vi "Configure Digital Alarm Parameters.vi"(0 "VISA resource name":refnum<visa-resource-name>, 1 "Alarm Number (1)":u16=1 min=1 max=8, 2 "Unit Address (1)":u8=1, 5 "Latching Mode (0: No Latch)":u16(ring)=1 items=["No Latch", "Automatic Latching", "Manual Latching", "Event Latching"], 7 "Priority (1: Low Priority)":u8(ring)=1 items=["Low Priority"=1, "Medium Priority"=2, "High Priority"=3], 9 "Display Delay (0)":u32 max=1800000000, 11 "error in (no error)":errorcluster, 12 "Alarm Inhibit  (False: Disable)":bool, 13 "Alarm Blocking Mode (False: Disable)":bool) -> (4 "VISA resource name out":refnum<visa-resource-name>, 15 "error out":errorcluster)   [LabVIEW 2014, in "Eurotherm 35xx Series.lvlib"]
doc: "This VI Configure parameters of selected digital alarm."
uses:
  <instrlib>/Eurotherm 35xx Series/Eurotherm 35xx Series.lvlib
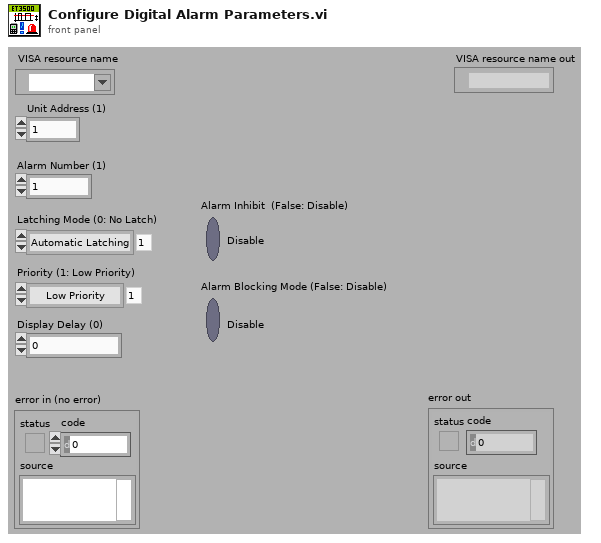
[diagram p1: front panel]
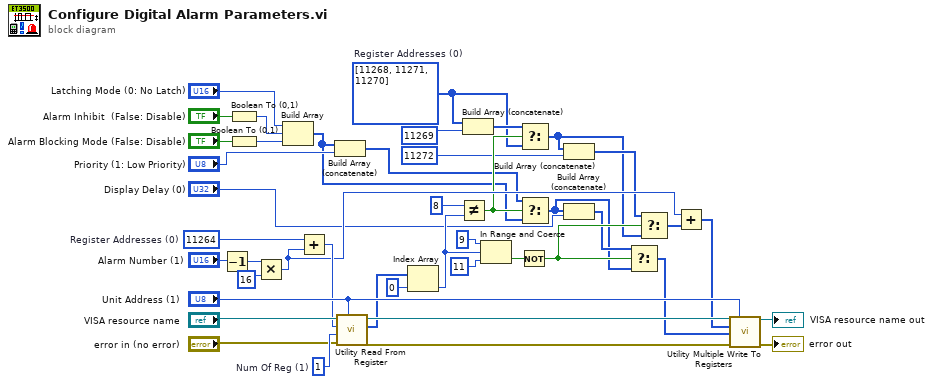
[diagram p0: block diagram]
diagram:
  w9 = u16[] [11268, 11271, 11270]  # Register Addresses (0)
  w34 = u16 1  # Num Of Reg (1)
  w40 = 11264  # Register Addresses (0)
  n1 = Decrement(x="Alarm Number (1)") -> (x-1=w42:u16)
  n2 = Boolean To (0,1)(Boolean="Alarm Inhibit  (False: Disable)") -> (0, 1=w24:i16)
  n3 = Boolean To (0,1)(Boolean="Alarm Blocking Mode (False: Disable)") -> (0, 1=w23:i16)
  n4 = Multiply(x=w42, y=u16 16) -> (x*y=w18:u16)
  n5 = Build Array("Latching Mode (0: No Latch)", w24, w23) -> (w7:u16[])
  n6 = Add(x=w40, y=w18) -> (x+y=w35:i32)
  n7 = Build Array (concatenate)(w7, "Priority (1: Low Priority)") -> (w8:u16[])
  n8 = call <instrlib>:"Utility Read From Register.vi"("Unit Address (1)"="Unit Address (1)", "error in (no error)"="error in (no error)", "Num Of Reg (1)"=w34, "Register Address (0)"=w35, "VISA resource name"="VISA resource name") -> ("error out"=w31:errorcluster, "Data"=w30:i16[], "VISA resource name out"=w32:refnum<visa-resource-name>)  [unwired: 4 in]
  n9 = Index Array(array=w30, index=0) -> (element=w12:i16)
  n10 = Not Equal?(x=u16 8, y=w12) -> (x != y?=w11:bool)
  n11 = Build Array (concatenate)(w9, 11269 ("y")) -> (w10:i32[])
  n12 = In Range and Coerce(upper limit=i16 9, x=w12, lower limit=i16 11) -> (In Range?=w15:bool)  [unwired: 1 out]
  n13 = Not(x=w15) -> (.not. x?=w14:bool)
  n14 = Select(t=w10, s=w11, f=w9) -> (s? t:f=w1:i32[])
  n15 = Select(t=w8, s=w11, f=w7) -> (s? t:f=w2:u16[])
  n16 = Build Array (concatenate)(w1, 11272 ("y")) -> (w4:i32[])
  n17 = Build Array (concatenate)(w2, "Display Delay (0)") -> (w3:u32[])
  n18 = Select(t=w3, s=w14, f=w2) -> (s? t:f=w21:u32[])
  n19 = Select(t=w4, s=w14, f=w1) -> (s? t:f=w20:i32[])
  n20 = Add(x=w18, y=w20) -> (x+y=w19:i32[])
  n21 = call <instrlib>:"Utility Multiple Write To Registers.vi"("VISA resource name"=w32, "Unit Address (1)"="Unit Address (1)", "Registers Addresses (0)"=w19, "Data (0)"=w21, "error in (no error)"=w31) -> ("VISA resource name out"=→"VISA resource name out":refnum<visa-resource-name>, "error out"=→"error out":errorcluster)  [unwired: 9 in]
